vi "Read Private Key.vi"(8 "error in (no error)":errorcluster, 11 "SSL Server Context in":refnum<class "SSL Server Context.lvclass">) -> (0 "error out":errorcluster, 2 "Private Key":path, 3 "SSL Server Context out":refnum<class "SSL Server Context.lvclass">)   [LabVIEW 2013, in "OpenSSL Socket.lvlib" / "SSL Server Context.lvclass"]
uses:
  SSL Server Context.lvclass
  SSL Server Context.lvclass/SSL Server Context.ctl
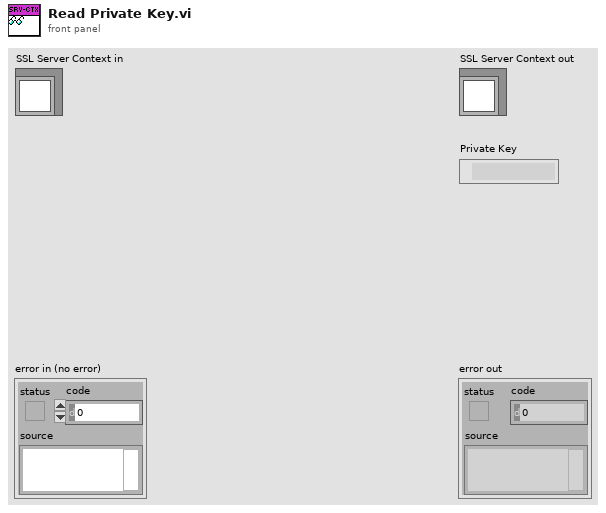
[diagram p1: front panel]
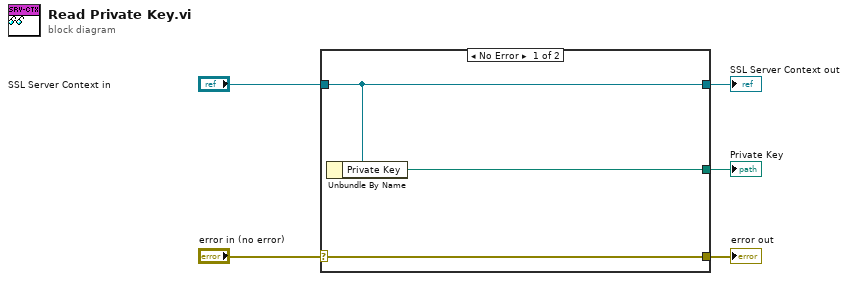
[diagram p0: block diagram]
diagram:
  n1 = case shown="No Error" "error in (no error)" {
    selector: "error in (no error)" -> [w8 w9]
    tunnel: [w8 w9] -> w4
    tunnel: [w7 w10] -> w2
    tunnel: "SSL Server Context in" -> [w7 w10]
    tunnel: [w6 _] -> w1
    frame No Error {
      n2 = Unbundle By Name(w7) -> ("Private Key"=w6:path)
    }
    frame Error {
    }
  }
  "error out" <- w4
  "SSL Server Context out" <- w2
  "Private Key" <- w1
